vi "FindCloseTagByName__NIMOD.vi"(6 "offset (0)":i32, 9 "max offset":i32, 10 "close Tag":string, 11 "string":string) -> (2 "match close tag":string, 4 "offset past close tag":i32)   [LabVIEW 2011]
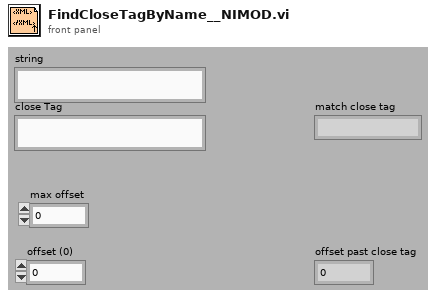
[diagram p1: front panel]
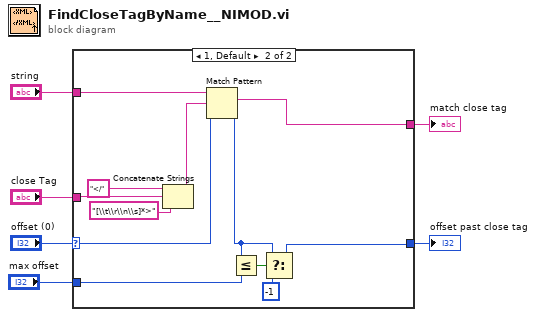
[diagram p0: block diagram]
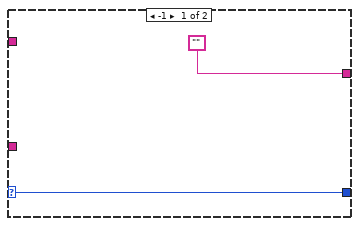
[diagram p2: hidden frame]
diagram:
  n1 = case shown="1, Default" "offset (0)" {
    selector: "offset (0)" -> [w8 w10]
    tunnel: "string" -> [_ w20]
    tunnel: "close Tag" -> [_ w17]
    tunnel: ["" w19] -> w4
    tunnel: [w8 w11] -> w3
    tunnel: "max offset" -> [_ w9]
    frame -1 {
    }
    frame 1, Default {
      n2 = Concatenate Strings("</" ("string"), w17, "[\\t\\r\\n\\s]*>" ("regular expression")) -> (w16:string)
      n3 = Match Pattern(string=w20, regular expression=w16, offset (0)=w10) -> (match substring=w19:string, offset past match=w12:i32)  [unwired: 2 out]
      n4 = Less Or Equal?(x=w12, y=w9) -> (x <= y?=w13:bool)
      n5 = Select(t=w12, s=w13, f=-1) -> (s? t:f=w11:i32)
    }
  }
  "match close tag" <- w4
  "offset past close tag" <- w3
